vi "struct_ads_vol_piStar_pyxgTpsatRhoM.vi"(0 "Reference working pair (Input)":i64, 1 "Molar fraction of refrigerant in adsorbed phase in mol/mol (Input)":dbl, 2 "Molar fraction of refrigerant in vapor phase in mol/mol (Input)":dbl, 3 "Total pressure of vapor phase in Pa (Input)":dbl, 5 "Temperature in K (Input)":dbl, 7 "Activity coefficient of refrigerant in adsorbed phase (Input)":dbl, 9 "Saturation vapor pressure in Pa (Input)":dbl, 11 "Error (Input)":errorcluster, 12 "Density of adsorpt in kg/m3 (Input)":dbl, 13 "Molar mass of refrigerant M in kg/mol (Input)":dbl) -> (4 "Reduced spreading pressure in kg/mol (Output)":dbl, 15 "Error (Output)":errorcluster caption="Error(Output)")   [LabVIEW 2017]
doc: "ads_vol_piStar_pyxgTpsatRhoM:\n * -----------------------------\n *\n * Calculates reduced spreading pressure in kg/mol depending on equilibrium\n * pressure p in Pa, molar fraction of refrigerant in vapor phase in mol/mol,\n * molar fraction of refrigerant in adsorbed phase in mol/mol, activity\n * coefficient of refrigerant in adsorbed phase, equilibrium temperature T in K,\n * saturation pressure p_Sat in Pa and density of adsorpt rho in kg/m³ and molar\n * mass of refrigerant M in kg/mol. The reduced spreading pressure is defined as\n * follows:\n *\n * piStar = A * pi / (R * T * m_sorbent) = 1 / M *\n * Integral_0^p0{w(p,T) / p * dp}\n *\n * where p0 = p_total*y / (gamma*x)\n *\n * Parameters:\n * -----------\n * double p_total_Pa:\n * Total pressure of vapor phase in Pa.\n * double y_molmol:\n * Molar fraction of refrigerant in vapor phase in mol/mol.\n * double x_molmol:\n * Molar fraction of refrigerant in adsorbed phase in mol/mol.\n * double gamma:\n * Activity coefficient of refrigerant in adsorbed phase.\n * double T_K:\n * Equilibrium temperature in K.\n * double p_sat_Pa:\n * Saturation pressure in Pa.\n * double rho_kgm3:\n * Density of adsorpt in kg/m³.\n * double M_kgmol:\n * Molar mass of refrigerant M in kg/mol.\n * struct *WorkingPair:\n * Pointer of WorkingPair-struct.\n *\n * Returns:\n * --------\n * double:\n * Reduced spreading pressure in kg/mol.\n *\n * Remarks:\n * --------\n * This function is only valid for isotherm models based on the volumetric\n * approach.\n *\n * History:\n * --------\n * 07/13/2021, by Jannik Driesel (supervised by Mirko Engelpracht):\n * First implementation."
uses:
  data/win32bit/libsorpPropLib.dll
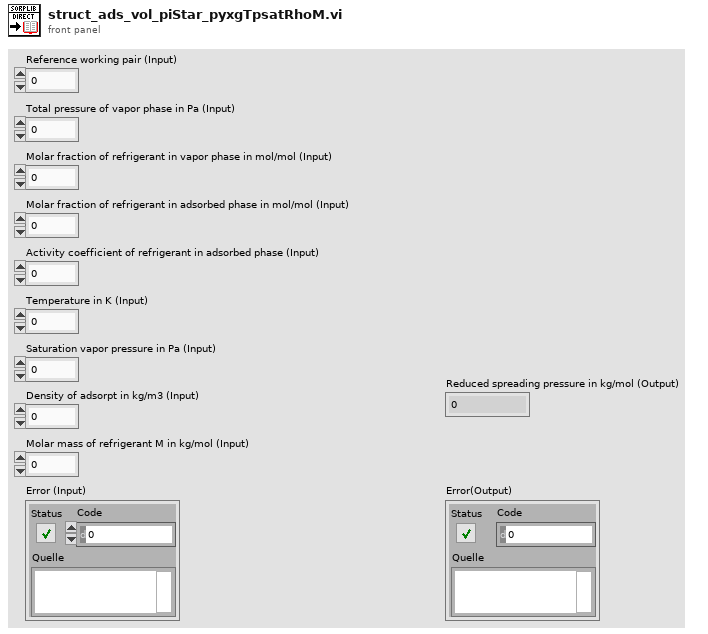
[diagram p1: front panel]
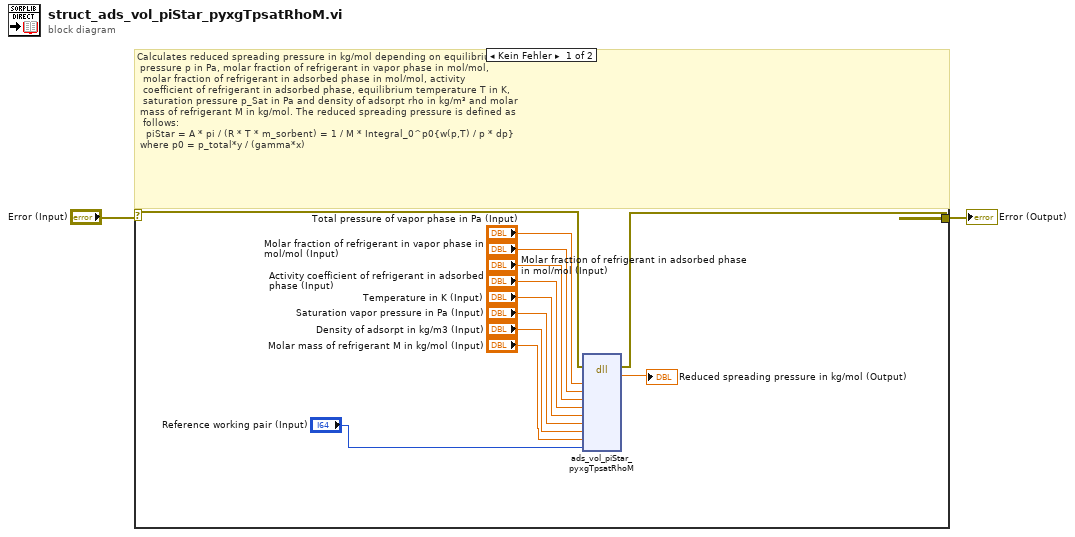
[diagram p0: block diagram]
diagram:
  n1 = case shown="Kein Fehler" "Error (Input)" {
    selector: "Error (Input)" -> [w13 w15]
    tunnel: [w12 w15] -> w1
    frame No Error {
      # "Calculates reduced spreading pressure in kg/mol depending on equilibrium\n pressure p in Pa, molar fraction of refrigerant in vapor phase in mol/mol,\n  molar fraction of refrigerant in adsorbed phase in mol/mol, activity\n  coefficient of refrigerant in adsorbed phase, equilibrium temperature T in K,\n  saturation pressure p_Sat in Pa and density of adsorpt rho in kg/m³ and molar\n mass of refrigerant M in kg/mol. The reduced spreading pressure is defined as\n  follows:\n  \tpiStar = A * pi / (R * T * m_sorbent) = 1 / M *\tIntegral_0^p0{w(p,T) / p * dp}\n where p0 = p_total*y / (gamma*x)"
      n2 = dll-call lib="D:/Driesel/SorpLibLocal/LabVIEW_wrapper/data/win32bit/libsorpPropLib.dll" fn="ads_vol_piStar_pyxgTpsatRhoM"(error in=w13, "p_total_Pa"="Total pressure of vapor phase in Pa (Input)", "y_molmol"="Molar fraction of refrigerant in vapor phase in mol/mol (Input)", "x_molmol"="Molar fraction of refrigerant in adsorbed phase in mol/mol (Input)", "gamma"="Activity coefficient of refrigerant in adsorbed phase (Input)", "T_K"="Temperature in K (Input)", "p_sat_Pa"="Saturation vapor pressure in Pa (Input)", "rho_kgm3"="Density of adsorpt in kg/m3 (Input)", "M_kgmol"="Molar mass of refrigerant M in kg/mol (Input)", "workingPair"="Reference working pair (Input)") -> (error out=w12:errorcluster, "piStar_kgmol"=→"Reduced spreading pressure in kg/mol (Output)":dbl)  [unwired: 11 in, 1 out]
    }
    frame Error {
      # "Error - No calculations"
    }
  }
  "Error (Output)" <- w1
